vi "TDC_ILA_use.vi"() -> ()   [LabVIEW 2017]
panel:
  out "error out 2":errorcluster
  in  "String":string
  in  "ILA":bool=TRUE
  in  "address":string="10.3.173.11"
  in  "error in (no error)":errorcluster
  out "error out":errorcluster
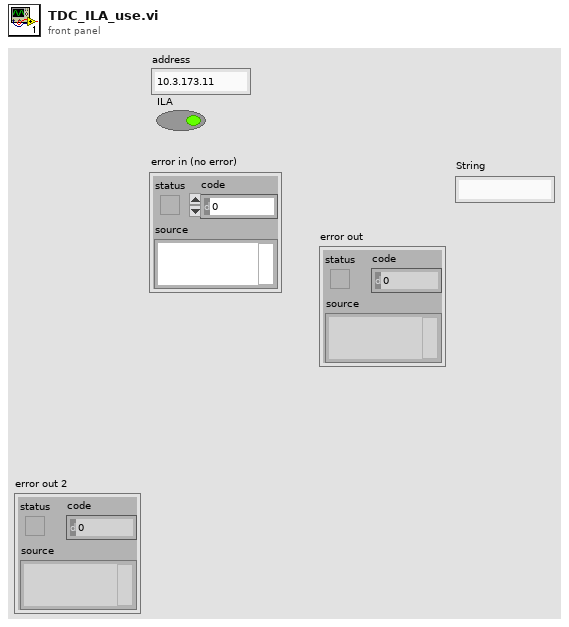
[diagram p1: front panel]
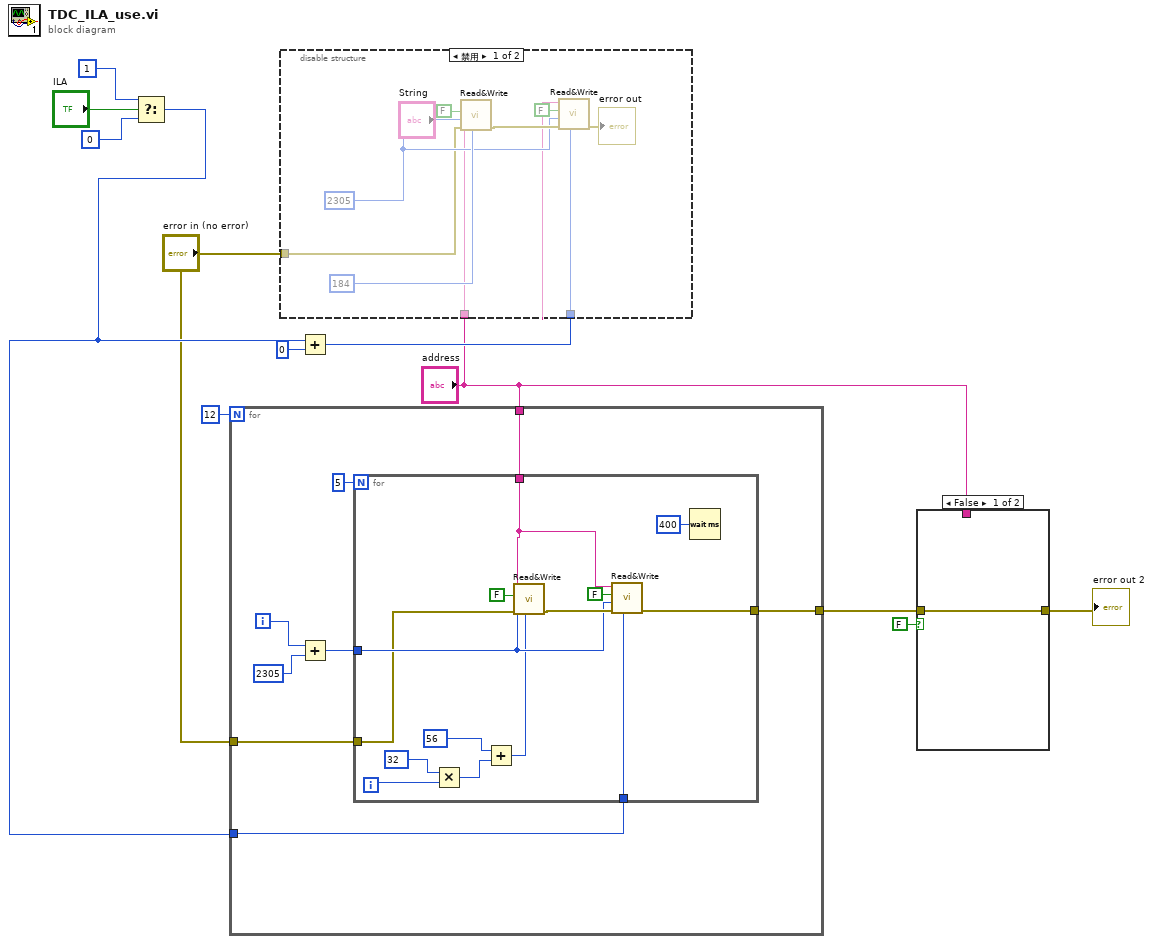
[diagram p0: block diagram]
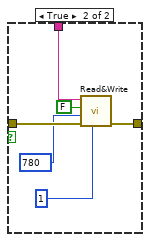
[diagram p2: hidden frame]
diagram:
  n1 = Select(t=u8 1 ("In 3"), s="ILA", f=u8 0 ("In 3")) -> (s? t:f=w6:u8)
  n2 = for {
    N: 12 -> [_]
    tunnel: "error in (no error)" -> [w16]
    tunnel: "address" -> [w15]
    tunnel: w6 -> [w14]
    tunnel: [w13] -> w4
    i -> [w18]
    n3 = Add(x=w18, y=u32 2305 ("Address")) -> (x+y=w19:u32)
    n4 = for {
      N: 5 -> [_]
      tunnel: w14 -> [w31]
      tunnel: w19 -> [w30]
      tunnel: w16 -> [w24]
      tunnel: w15 -> [w23]
      tunnel: [w22] -> w13
      i -> [w28]
      n5 = Multiply(x=u8 32 ("In"), y=w28) -> (x*y=w26:i32)
      n6 = Add(x=u8 56 ("In"), y=w26) -> (x+y=w25:i32)
      n7 = call "Read&Write.vi"("In"=w25, "error in (no error)"=w24, "Address"=w30, "Read (TRUE)"=FALSE, "address"=w23) -> ("error out"=w34:errorcluster)  [unwired: 5 in, 1 out]
      n8 = call "Read&Write.vi"("In"=w31, "error in (no error)"=w34, "Address"=w30, "Read (TRUE)"=FALSE, "address"=w23) -> ("error out"=w22:errorcluster)  [unwired: 5 in, 1 out]
      n9 = Wait (ms)(milliseconds to wait=u32 400) -> ()  [unwired: 1 out]
    }
  }
  n10 = Add(x=w6, y=u8 0) -> (x+y=w10:u8)
  n11 = disable-structure shown="禁用" {
    disable-tunnel: w10 -> [w37 _]
    disable-tunnel: "address" -> [w36 _]
    disable-tunnel: "error in (no error)" -> [w35 _]
    frame Disabled {
      w38 = u32 2305 ("Address")
      n12 = call "Read&Write.vi"("In"=u8 184, "error in (no error)"=w35, "Address"=w38, "Read (TRUE)"=FALSE, "address"=w36) -> ("error out"=w43:errorcluster)  [unwired: 5 in, 1 out]
      n13 = call "Read&Write.vi"("In"=w37, "error in (no error)"=w43, "Address"=w38, "Read (TRUE)"=FALSE, "address"=w36) -> ("error out"=→"error out":errorcluster)  [unwired: 5 in, 1 out]
    }
    frame Enabled {
    }
  }
  n14 = case shown="False" FALSE {
    tunnel: w4 -> [w44 w49]
    tunnel: "address" -> [_ w47]
    tunnel: [w44 w45] -> w2
    frame False {
    }
    frame True {
      n15 = call "Read&Write.vi"("In"=u8 1, "error in (no error)"=w49, "Address"=u32 780, "Read (TRUE)"=FALSE, "address"=w47) -> ("error out"=w45:errorcluster)  [unwired: 5 in, 1 out]
    }
  }
  "error out 2" <- w2
